vi "nmea.vi"(8 "ecef ref":dbl[](array[numeric]) format="%#_19f", 11 "NMEA":string) -> (0 "output":dbl[](array[numeric]) format="%#_19f", 3 "type":u32)   [LabVIEW 2015]
uses:
  <vilib>/Analysis/Matrix/Numeric/Conversions/Array To Matrix - RA.vi
  <vilib>/Analysis/Matrix/Numeric/Conversions/Array To Matrix - RA2.vi
  <vilib>/Analysis/Matrix/Numeric/Multiply/Multiply - RM,RM.vi
  <vilib>/Analysis/Matrix/Numeric/Conversions/Matrix To Array - RM.vi
  <vilib>/Analysis/Matrix/NI_Matrix.lvlib
panel:
  out "trk gnd":dbl
  out "speed":dbl
  out "sol stat":i16
  out "ms rmc":dbl format="%#_6f"
  out "lat rmc":dbl format="%#_12f"
  out "lon rmc":dbl format="%#_12f"
  out "ecef":dbl[](array[numeric]) format="%#_19f"
  out "DCM(ecef2lcc)":dbl[][](array[numeric])
  out "diff_age":i32
  out "hgt":i32
  out "dev":dbl
  out "#SV":i32
  out "pos type":i32
  out "lon":dbl format="%#_12f"
  out "lat":dbl format="%#_12f"
  out "ms":dbl format="%#_6f"
  out "chksum":bool
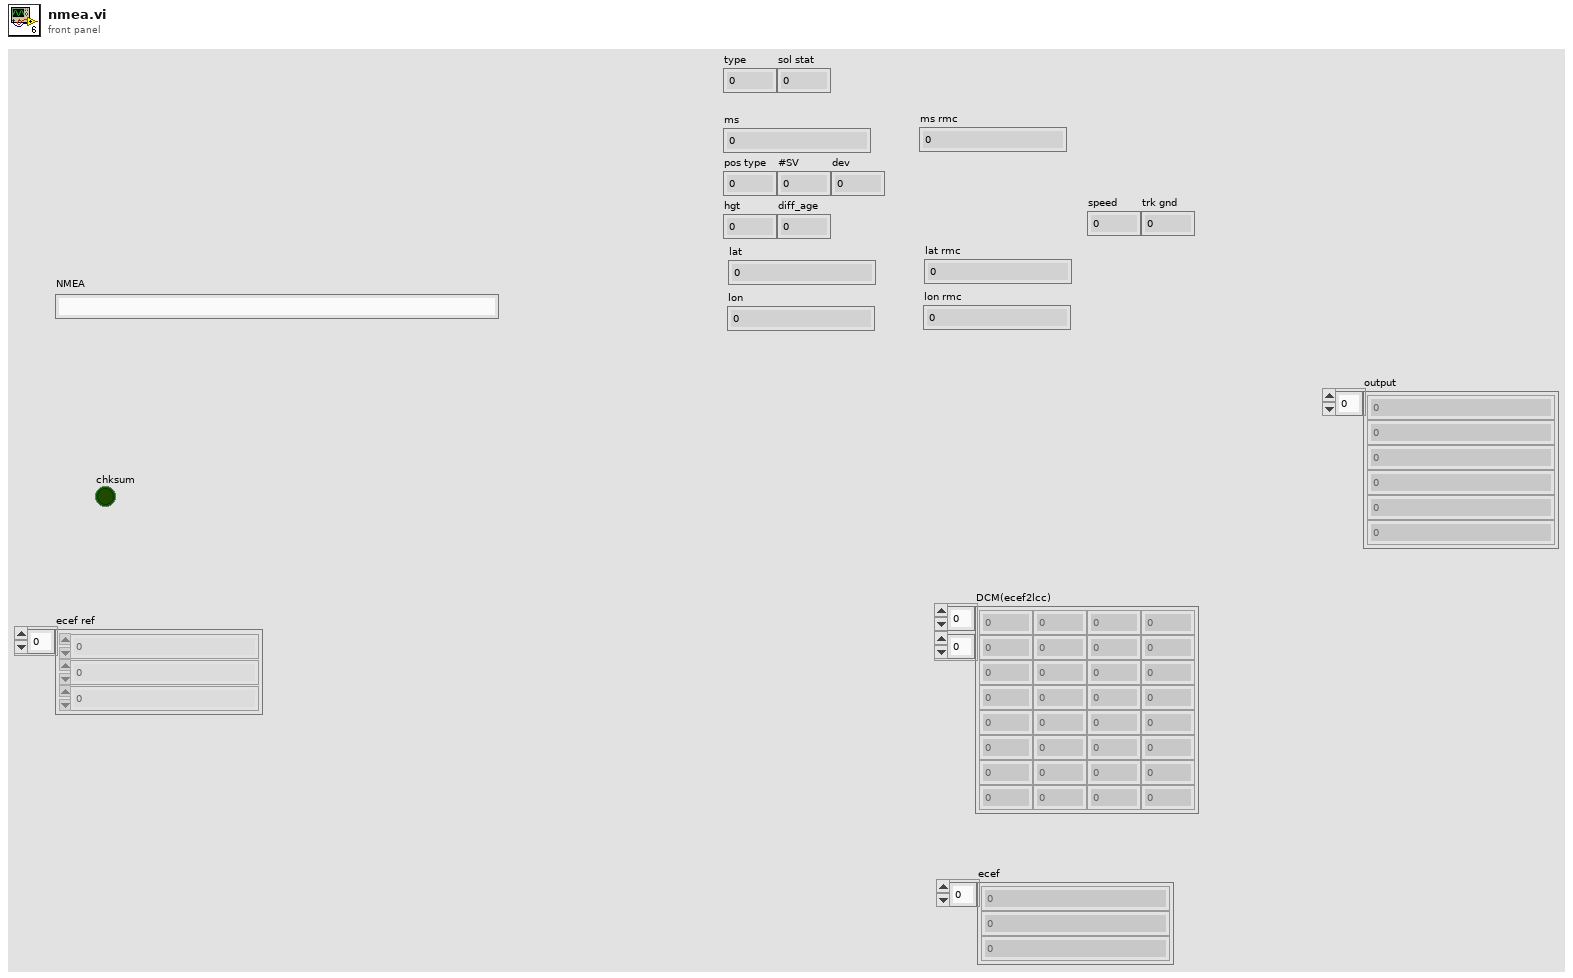
[diagram p1: front panel]
types:
  T1 = typedef "NI_Matrix.lvlib/RealMatrix.ctl" = dbl[][]
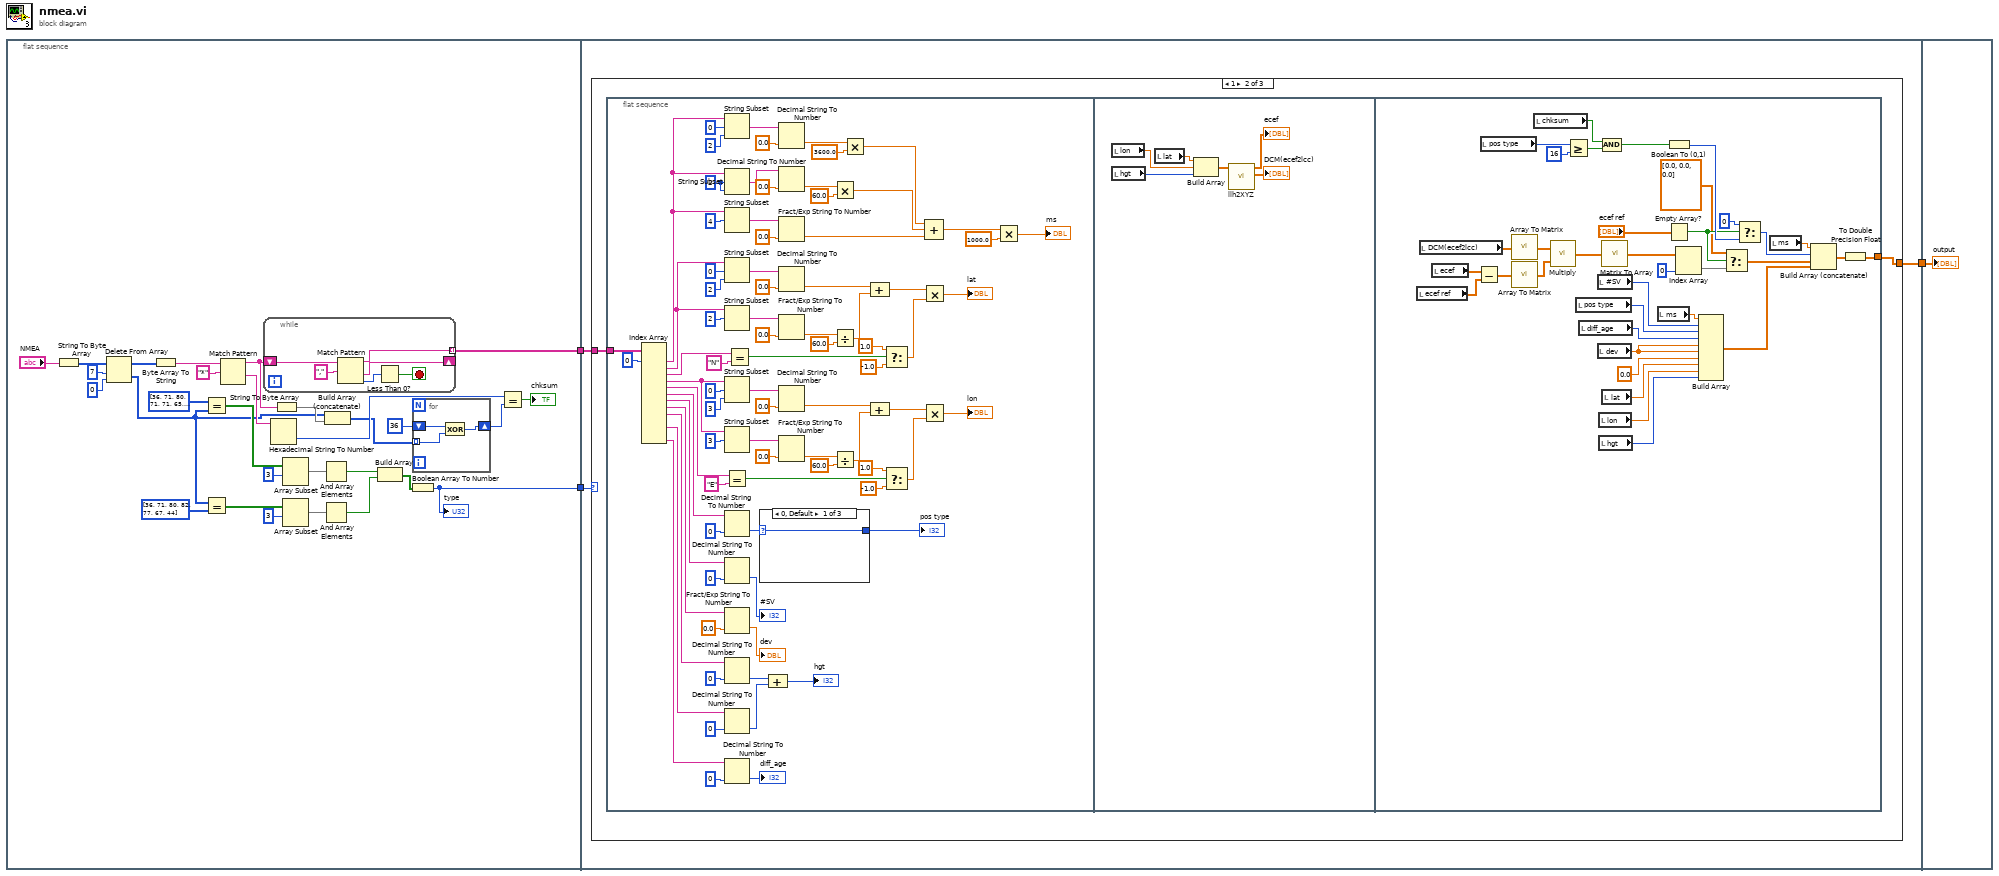
[diagram p0: block diagram]
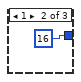
[diagram p3: hidden frame]
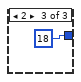
[diagram p4: hidden frame]
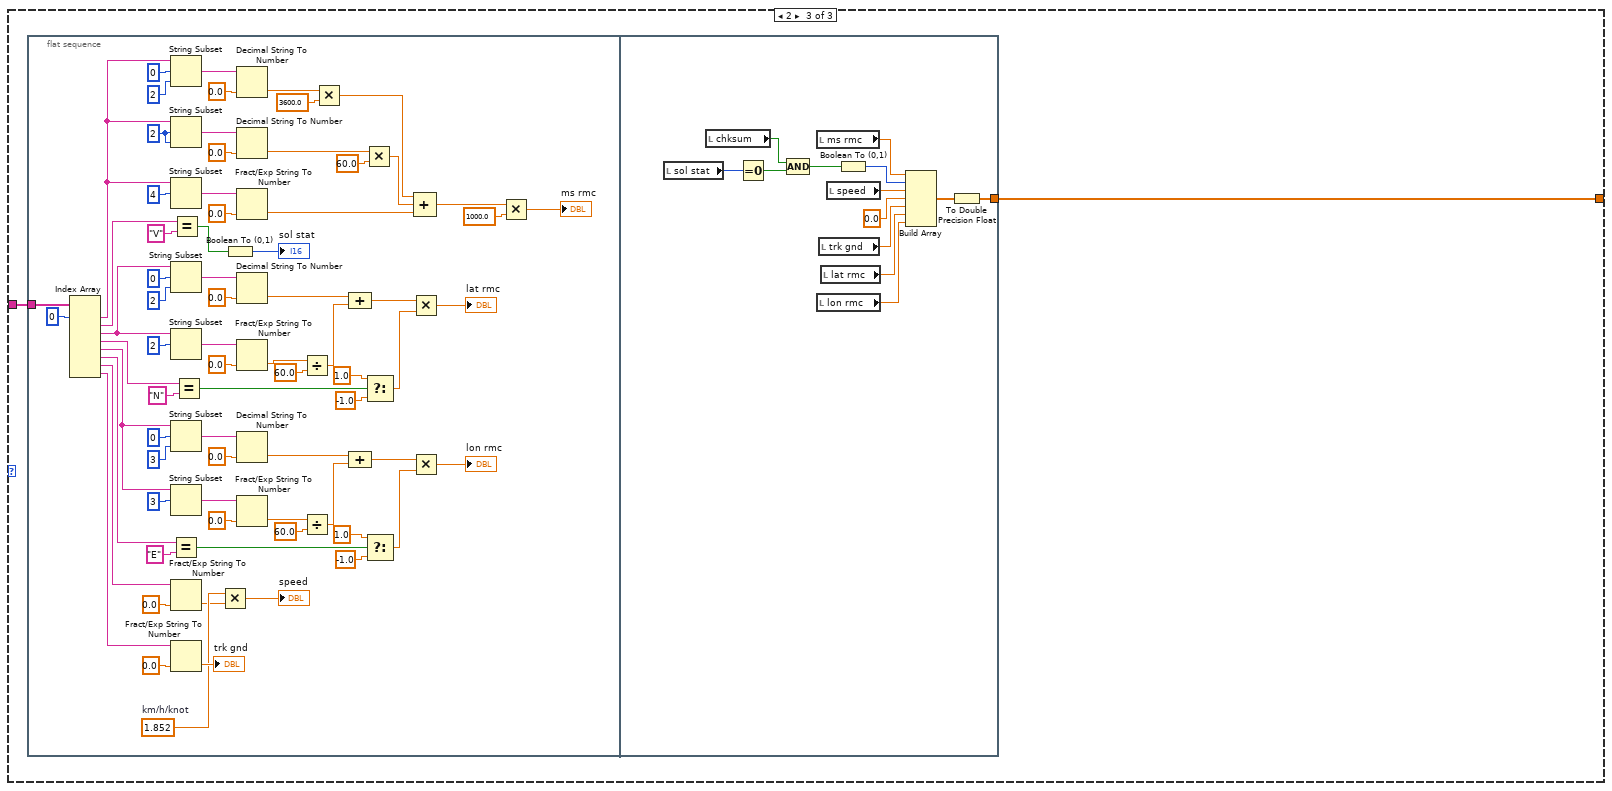
[diagram p5: hidden frame]
diagram:
  n1 = flat-sequence {
    tunnel: [w15] -> w3
    tunnel: [w14] -> w2
    tunnel: w3 -> [w44]
    tunnel: w2 -> [w43]
    tunnel: [w42] -> w1
    tunnel: w1 -> [w264]
    frame #0 {
      n2 = String To Byte Array(string="NMEA") -> (unsigned byte array=w32:u8[])
      n3 = Delete From Array(array=w32, length=7, index=0) -> (deleted portion=w4:u8[], array with subset deleted=w29:u8[])
      n4 = Byte Array To String(unsigned byte array=w29) -> (string=w26:string)
      n5 = Equal?(x=u8[] [36, 71, 80, 71, 71, 65, 44] ("gpgga"), y=w4) -> (x = y?=w13:bool[])
      n6 = Equal?(x=w4, y=u8[] [36, 71, 80, 82, 77, 67, 44] ("gprmc")) -> (x = y?=w9:bool[])
      n7 = Match Pattern(string=w26, regular expression="*") -> (before substring=w22:string, after substring=w21:string)  [unwired: 1 in, 2 out]
      n8 = while {
        shift-right: [w40] -> _
        shift-left: w22 -> [w41]
        tunnel: [w38] -> w15 mode=indexing
        stop <- w36 stop-if-true
        n9 = Match Pattern(string=w41, regular expression=",") -> (before substring=w38:string, after substring=w40:string, offset past match=w37:i32)  [unwired: 1 in, 1 out]
        n10 = Less Than 0?(x=w37) -> (x < 0?=w36:bool)
      }
      n11 = Hexadecimal String To Number(string=w21) -> (number=w18:u32)  [unwired: 2 in, 1 out]
      n12 = String To Byte Array(string=w22) -> (unsigned byte array=w6:u8[])
      n13 = Array Subset(array=w13, index=3) -> (w12:bool[])  [unwired: 1 in]
      n14 = Array Subset(array=w9, index=3) -> (w8:bool[])  [unwired: 1 in]
      n15 = And Array Elements(Boolean array=w12) -> (logical AND=w28:bool)
      n16 = And Array Elements(Boolean array=w8) -> (logical AND=w17:bool)
      n17 = Build Array (concatenate)(w4, w6) -> (w5:u8[])
      n18 = Build Array(w28, w17) -> (w27:bool[])
      n19 = Boolean Array To Number(Boolean array=w27) -> (number=w14:u32)
      "type" <- w14
      n20 = for {
        tunnel: w5 -> [w34] mode=indexing
        shift-right: [w33] -> w19
        shift-left: u8 36 -> [w35]
        n21 = Exclusive Or(1:w34, 2:w35) -> (0:w33:u8)
      }
      n22 = Equal?(x=w18, y=w19) -> (x = y?=→"chksum":bool)
    }
    frame #1 {
      n23 = case shown="1" w43 {
        tunnel: w44 -> [_ w46 w175]
        tunnel: [_ w45 w174] -> w42
        frame 0, Default {
        }
        frame 1 {
          n24 = flat-sequence {
            tunnel: w46 -> [w129]
            tunnel: [w139] -> w45
            frame #0 {
              w125 = 2 ("length (rest)")
              n25 = Index Array(array=w129, index #1=0 ("index")) -> (element #1=w96:string, element #2=w95:string, element #3=w94:string, element #4=w68:string, element #5=w67:string, element #6=w66:string, element #7=w61:string, element #8=w58:string, element #9=w55:string, element #11=w53:string, element #13=w48:string)  [unwired: 12 in, 2 out]
              n26 = String Subset(string=w96, offset (0)=0, length (rest)=2 ("length (rest)")) -> (substring=w123:string)
              n27 = String Subset(string=w96, offset (0)=w125, length (rest)=w125) -> (substring=w117:string)
              n28 = String Subset(string=w96, offset (0)=4) -> (substring=w113:string)  [unwired: 1 in]
              n29 = String Subset(string=w95, offset (0)=0, length (rest)=2 ("length (rest)")) -> (substring=w104:string)
              n30 = String Subset(string=w95, offset (0)=2) -> (substring=w106:string)  [unwired: 1 in]
              n31 = String Subset(string=w68, offset (0)=0, length (rest)=3 ("length (rest)")) -> (substring=w72:string)
              n32 = String Subset(string=w68, offset (0)=3) -> (substring=w70:string)  [unwired: 1 in]
              n33 = Equal?(x=w67, y="E") -> (x = y?=w81:bool)
              n34 = Decimal String To Number(string=w66, default (0L)=0 ("default (0 I32)")) -> (number=w64:i32)  [unwired: 1 in, 1 out]
              n35 = Decimal String To Number(string=w61, default (0L)=0 ("default (0 I32)")) -> (number=→"#SV":i32)  [unwired: 1 in, 1 out]
              n36 = Fract/Exp String To Number(string=w58, default (0 dbl)=0.0 ("default (0 I32)")) -> (number=→"dev":dbl)  [unwired: 2 in, 1 out]
              n37 = Decimal String To Number(string=w55, default (0L)=0 ("default (0 I32)")) -> (number=w52:i32)  [unwired: 1 in, 1 out]
              n38 = Decimal String To Number(string=w53, default (0L)=0 ("default (0 I32)")) -> (number=w51:i32)  [unwired: 1 in, 1 out]
              n39 = Decimal String To Number(string=w48, default (0L)=0 ("default (0 I32)")) -> (number=→"diff_age":i32)  [unwired: 1 in, 1 out]
              n40 = Equal?(x=w94, y="N") -> (x = y?=w92:bool)
              n41 = case shown="0, Default" w64 {
                selector: w64 -> [w130 _ _]
                tunnel: [w130 16 18] -> w63
                frame 0, Default {
                }
                frame 1 {
                }
                frame 2 {
                }
              }
              "pos type" <- w63
              n42 = Compound Arithmetic op=ADD(w52, w51) -> (→"hgt":i32)
              n43 = Decimal String To Number(string=w123, default (0L)=0.0 ("default (0 I32)")) -> (number=w122:dbl)  [unwired: 1 in, 1 out]
              n44 = Decimal String To Number(string=w117, default (0L)=0.0 ("default (0 I32)")) -> (number=w118:dbl)  [unwired: 1 in, 1 out]
              n45 = Fract/Exp String To Number(string=w113, default (0 dbl)=0.0 ("default (0 I32)")) -> (number=w111:dbl)  [unwired: 2 in, 1 out]
              n46 = Decimal String To Number(string=w104, default (0L)=0.0 ("default (0 I32)")) -> (number=w100:dbl)  [unwired: 1 in, 1 out]
              n47 = Fract/Exp String To Number(string=w106, default (0 dbl)=0.0 ("default (0 I32)")) -> (number=w99:dbl)  [unwired: 2 in, 1 out]
              n48 = Decimal String To Number(string=w72, default (0L)=0.0 ("default (0 I32)")) -> (number=w76:dbl)  [unwired: 1 in, 1 out]
              n49 = Fract/Exp String To Number(string=w70, default (0 dbl)=0.0 ("default (0 I32)")) -> (number=w77:dbl)  [unwired: 2 in, 1 out]
              n50 = Multiply(x=w118, y=60.0) -> (x*y=w114:dbl)
              n51 = Divide(x=w99, y=60.0) -> (x/y=w97:dbl)
              n52 = Divide(x=w77, y=60.0) -> (x/y=w79:dbl)
              n53 = Multiply(x=w122, y=3600.0) -> (x*y=w115:dbl)
              n54 = Compound Arithmetic op=ADD(w100, w97) -> (w89:dbl)
              n55 = Compound Arithmetic op=ADD(w76, w79) -> (w84:dbl)
              n56 = Select(t=1.0, s=w92, f=-1.0) -> (s? t:f=w88:dbl)
              n57 = Select(t=1.0, s=w81, f=-1.0) -> (s? t:f=w85:dbl)
              n58 = Multiply(x=w89, y=w88) -> (x*y=→"lat":dbl)
              n59 = Multiply(x=w84, y=w85) -> (x*y=→"lon":dbl)
              n60 = Compound Arithmetic op=ADD(w115, w114, w111) -> (w110:dbl)
              n61 = Multiply(x=w110, y=1000.0) -> (x*y=→"ms":dbl)
            }
            frame #1 {
              n62 = local read "lon"() -> (w137:dbl)
              n63 = local read "hgt"() -> (w136:i32)
              n64 = local read "lat"() -> (w138:dbl)
              n65 = Build Array(w138, w137, w136) -> (w135:dbl[])
              n66 = call "llh2XYZ.vi"("llh"=w135) -> ("DCM(ecef2lcc)"=→"DCM(ecef2lcc)":dbl[][], "ecef"=→"ecef":dbl[])  [unwired: 7 in]
            }
            frame #2 {
              n67 = local read "ecef ref"() -> (w155:dbl[])
              n68 = local read "DCM(ecef2lcc)"() -> (w156:dbl[][])
              n69 = local read "ecef"() -> (w154:dbl[])
              n70 = Subtract(x=w154, y=w155) -> (x-y=w158:dbl[])
              n71 = local read "pos type"() -> (w149:i32)
              n72 = call-poly <vilib>:"Array To Matrix.vi"("Real 2D Array"=w156) -> ("Real Matrix"=w157:T1)
              n73 = call-poly <vilib>:"Array To Matrix.vi"("Real 1D Array"=w158) -> ("Real Matrix (Column Vector)"=w159:T1)
              n74 = local read "chksum"() -> (w148:bool)
              n75 = call-poly <vilib>:"Multiply.vi"("Real Matrix B"=w159, "Real Matrix A"=w157) -> ("A * B"=w160:T1)
              n76 = Greater Or Equal?(x=w149, y=u32 16) -> (x >= y?=w165:bool)
              n77 = local read "pos type"() -> (w146:i32)
              n78 = local read "diff_age"() -> (w145:i32)
              n79 = local read "#SV"() -> (w147:i32)
              n80 = local read "dev"() -> (w144:dbl)
              n81 = local read "lon"() -> (w141:dbl)
              n82 = local read "hgt"() -> (w140:i32)
              n83 = call-poly <vilib>:"Matrix To Array.vi"("Real Matrix"=w160) -> ("Real 2D Array"=w161:dbl[][])
              n84 = local read "lat"() -> (w142:dbl)
              n85 = Compound Arithmetic op=AND(w148, w165) -> (w166:bool)
              n86 = local read "ms"() -> (w150:dbl)
              n87 = Boolean To (0,1)(Boolean=w166) -> (0, 1=w171:i16)
              n88 = Empty Array?(array="ecef ref") -> (empty?=w170:bool)
              n89 = Index Array(array=w161, index (col)=0 ("disabled index (col)")) -> (element=w168:dbl[])  [unwired: 1 in]
              n90 = Build Array(w150, w147, w146, w145, w144, w144, 0.0 ("element"), w142, w141, w140) -> (w167:dbl[])
              n91 = Select(t=dbl[] [0.0, 0.0, 0.0] ("subarray"), s=w170, f=w168) -> (s? t:f=w169:dbl[])
              n92 = Select(t=i16 0, s=w170, f=w171) -> (s? t:f=w172:i16)
              n93 = local read "ms"() -> (w151:dbl)
              n94 = Build Array (concatenate)(w151, w172, w169, w167) -> (w163:dbl[])
              n95 = To Double Precision Float(number=w163) -> (double precision float=w139:dbl[])
            }
          }
        }
        frame 2 {
          n96 = flat-sequence {
            tunnel: w175 -> [w250]
            tunnel: [w253] -> w174
            frame #0 {
              w177 = 1.852  # km/h/knot
              w247 = 2 ("length (rest)")
              n97 = Index Array(array=w250, index #1=0 ("index")) -> (element #1=w189:string, element #2=w187:string, element #3=w218:string, element #4=w217:string, element #5=w191:string, element #6=w190:string, element #7=w183:string, element #8=w179:string)  [unwired: 7 in]
              n98 = String Subset(string=w189, offset (0)=0, length (rest)=2 ("length (rest)")) -> (substring=w245:string)
              n99 = String Subset(string=w189, offset (0)=w247, length (rest)=w247) -> (substring=w239:string)
              n100 = String Subset(string=w189, offset (0)=4) -> (substring=w235:string)  [unwired: 1 in]
              n101 = String Subset(string=w218, offset (0)=0, length (rest)=2 ("length (rest)")) -> (substring=w226:string)
              n102 = String Subset(string=w218, offset (0)=2) -> (substring=w228:string)  [unwired: 1 in]
              n103 = String Subset(string=w191, offset (0)=0, length (rest)=3 ("length (rest)")) -> (substring=w195:string)
              n104 = String Subset(string=w191, offset (0)=3) -> (substring=w193:string)  [unwired: 1 in]
              n105 = Equal?(x=w190, y="E") -> (x = y?=w204:bool)
              n106 = Fract/Exp String To Number(string=w183, default (0 dbl)=0.0 ("default (0 I32)")) -> (number=w176:dbl)  [unwired: 2 in, 1 out]
              n107 = Fract/Exp String To Number(string=w179, default (0 dbl)=0.0 ("default (0 I32)")) -> (number=→"trk gnd":dbl)  [unwired: 2 in, 1 out]
              n108 = Equal?(x=w187, y="V") -> (x = y?=w185:bool)
              n109 = Equal?(x=w217, y="N") -> (x = y?=w215:bool)
              n110 = Multiply(x=w177, y=w176) -> (x*y=→"speed":dbl)
              n111 = Boolean To (0,1)(Boolean=w185) -> (0, 1=→"sol stat":i16)
              n112 = Decimal String To Number(string=w245, default (0L)=0.0 ("default (0 I32)")) -> (number=w244:dbl)  [unwired: 1 in, 1 out]
              n113 = Decimal String To Number(string=w239, default (0L)=0.0 ("default (0 I32)")) -> (number=w240:dbl)  [unwired: 1 in, 1 out]
              n114 = Fract/Exp String To Number(string=w235, default (0 dbl)=0.0 ("default (0 I32)")) -> (number=w233:dbl)  [unwired: 2 in, 1 out]
              n115 = Decimal String To Number(string=w226, default (0L)=0.0 ("default (0 I32)")) -> (number=w222:dbl)  [unwired: 1 in, 1 out]
              n116 = Fract/Exp String To Number(string=w228, default (0 dbl)=0.0 ("default (0 I32)")) -> (number=w221:dbl)  [unwired: 2 in, 1 out]
              n117 = Decimal String To Number(string=w195, default (0L)=0.0 ("default (0 I32)")) -> (number=w199:dbl)  [unwired: 1 in, 1 out]
              n118 = Fract/Exp String To Number(string=w193, default (0 dbl)=0.0 ("default (0 I32)")) -> (number=w200:dbl)  [unwired: 2 in, 1 out]
              n119 = Divide(x=w221, y=60.0) -> (x/y=w219:dbl)
              n120 = Divide(x=w200, y=60.0) -> (x/y=w202:dbl)
              n121 = Multiply(x=w244, y=3600.0) -> (x*y=w237:dbl)
              n122 = Compound Arithmetic op=ADD(w222, w219) -> (w212:dbl)
              n123 = Compound Arithmetic op=ADD(w199, w202) -> (w207:dbl)
              n124 = Multiply(x=w240, y=60.0) -> (x*y=w236:dbl)
              n125 = Select(t=1.0, s=w215, f=-1.0) -> (s? t:f=w211:dbl)
              n126 = Select(t=1.0, s=w204, f=-1.0) -> (s? t:f=w208:dbl)
              n127 = Multiply(x=w212, y=w211) -> (x*y=→"lat rmc":dbl)
              n128 = Multiply(x=w207, y=w208) -> (x*y=→"lon rmc":dbl)
              n129 = Compound Arithmetic op=ADD(w237, w236, w233) -> (w232:dbl)
              n130 = Multiply(x=w232, y=1000.0) -> (x*y=→"ms rmc":dbl)
            }
            frame #1 {
              n131 = local read "sol stat"() -> (w257:i16)
              n132 = local read "chksum"() -> (w260:bool)
              n133 = Equal To 0?(x=w257) -> (x = 0?=w261:bool)
              n134 = Compound Arithmetic op=AND(w260, w261) -> (w262:bool)
              n135 = local read "ms rmc"() -> (w258:dbl)
              n136 = local read "lon rmc"() -> (w251:dbl)
              n137 = local read "trk gnd"() -> (w254:dbl)
              n138 = local read "lat rmc"() -> (w252:dbl)
              n139 = local read "speed"() -> (w256:dbl)
              n140 = Boolean To (0,1)(Boolean=w262) -> (0, 1=w263:i16)
              n141 = Build Array(w258, w263, w256, 0.0 ("element"), w254, w252, w251) -> (w259:dbl[])
              n142 = To Double Precision Float(number=w259) -> (double precision float=w253:dbl[])
            }
          }
        }
      }
    }
    frame #2 {
      "output" <- w264
    }
  }
